vi "Add Major and Minor Frames.vi"(8 "error in":errorcluster, 9 "minor frames":T1[](array[typedef]), 10 "major frames":T2[](array[typedef]), 11 "port in":T3 format="%.0x") -> (0 "error out":errorcluster, 3 "port out":T3 format="%.0x")   [LabVIEW 2020, in "AIM MIL-STD-1553 Scripting.lvlib"]
doc: "Adds all <b>major frames</b> and <b>minor frames</b> to the <b>port in</b> in the custom device system definition."
uses:
  AIM MIL-STD-1553 Scripting.lvlib
  <vilib>/NI VeriStand/Custom Device API/Custom Device API.lvlib
  Constants.vi
  <vilib>/NI VeriStand/Custom Device API/Set Item Property (String Array).vi
  <vilib>/NI VeriStand/Custom Device API/Custom Device Item Ref.ctl
  Shared/Major Frame Definition.ctl
  Shared/Minor Frame Definition.ctl
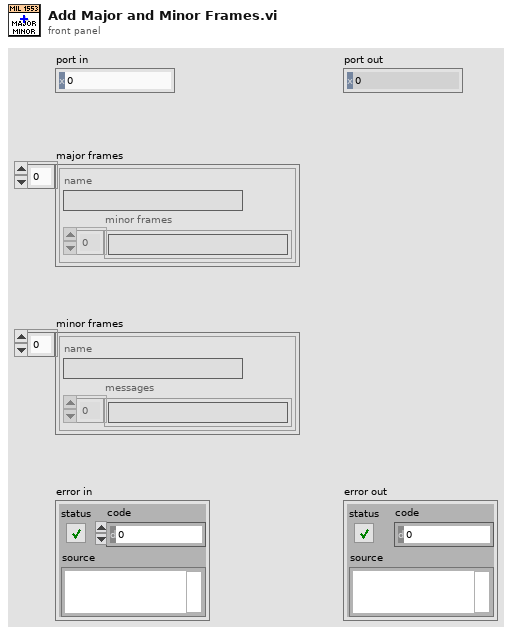
[diagram p1: front panel]
types:
  T1 = typedef "Minor Frame Definition.ctl" = cluster{"name":string, "messages":string[]}
  T2 = typedef "Major Frame Definition.ctl" = cluster{"name":string, "minor frames":string[]}
  T3 = typedef "Custom Device API.lvlib/Custom Device Item Ref.ctl" = u64
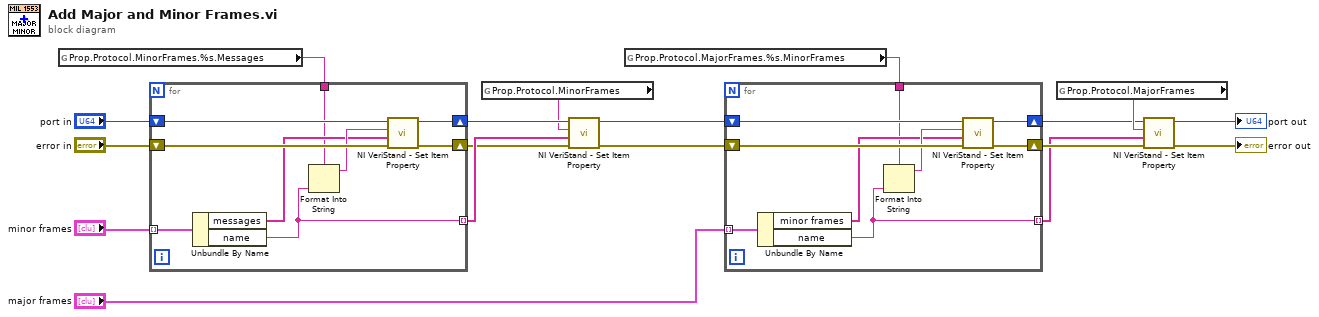
[diagram p0: block diagram]
diagram:
  n1 = global read "Constants.vi" "Prop.Protocol.MinorFrames.%s.Messages"() -> (w10:string)
  n2 = for {
    shift-right: [w24] -> w7
    shift-left: "error in" -> [w23]
    shift-right: [w25] -> w8
    shift-left: "port in" -> [w26]
    tunnel: "minor frames" -> [w27] mode=indexing
    tunnel: [w21] -> w9 mode=indexing
    tunnel: w10 -> [w19]
    n3 = Unbundle By Name(w27) -> ("messages"=w20:string[], "name"=w21:string)
    n4 = Format Into String(format string=w19, w21) -> (resulting string=w22:string)  [unwired: 2 in, 1 out]
    n5 = call-poly <vilib>:"NI VeriStand - Set Item Property.vi"("error in (no error)"=w23, "Value"=w20, "Property Name"=w22, "Item Ref in"=w26) -> ("error out"=w24:errorcluster, "Item Ref out"=w25:T3)  [unwired: 5 in, 1 out]
  }
  n6 = global read "Constants.vi" "Prop.Protocol.MinorFrames"() -> (w6:string)
  n7 = call-poly <vilib>:"NI VeriStand - Set Item Property.vi"("error in (no error)"=w7, "Value"=w9, "Property Name"=w6, "Item Ref in"=w8) -> ("error out"=w3:errorcluster, "Item Ref out"=w2:T3)  [unwired: 5 in, 1 out]
  n8 = global read "Constants.vi" "Prop.Protocol.MajorFrames.%s.MinorFrames"() -> (w11:string)
  n9 = for {
    shift-right: [w33] -> w16
    shift-left: w3 -> [w32]
    shift-right: [w34] -> w13
    shift-left: w2 -> [w35]
    tunnel: "major frames" -> [w36] mode=indexing
    tunnel: [w30] -> w12 mode=indexing
    tunnel: w11 -> [w28]
    n10 = Unbundle By Name(w36) -> ("minor frames"=w29:string[], "name"=w30:string)
    n11 = Format Into String(format string=w28, w30) -> (resulting string=w31:string)  [unwired: 2 in, 1 out]
    n12 = call-poly <vilib>:"NI VeriStand - Set Item Property.vi"("error in (no error)"=w32, "Value"=w29, "Property Name"=w31, "Item Ref in"=w35) -> ("error out"=w33:errorcluster, "Item Ref out"=w34:T3)  [unwired: 5 in, 1 out]
  }
  n13 = global read "Constants.vi" "Prop.Protocol.MajorFrames"() -> (w18:string)
  n14 = call-poly <vilib>:"NI VeriStand - Set Item Property.vi"("error in (no error)"=w16, "Value"=w12, "Property Name"=w18, "Item Ref in"=w13) -> ("error out"=→"error out":errorcluster, "Item Ref out"=→"port out":T3)  [unwired: 5 in, 1 out]
